vi "PPR_DRIVE_DASH_WRITE.vi"   [LabVIEW 2019]
uses:
  PPR_DRIVE_GLOBALS.vi
  <vilib>/Rock Robotics/Network Tables/NT Write Number.vi
  <vilib>/Rock Robotics/Network Tables/NT Write Numeric Array.vi
  <vilib>/Rock Robotics/WPI/ThirdParty/JAS_Junk/TrajLib/Trajectory_Library.lvlib
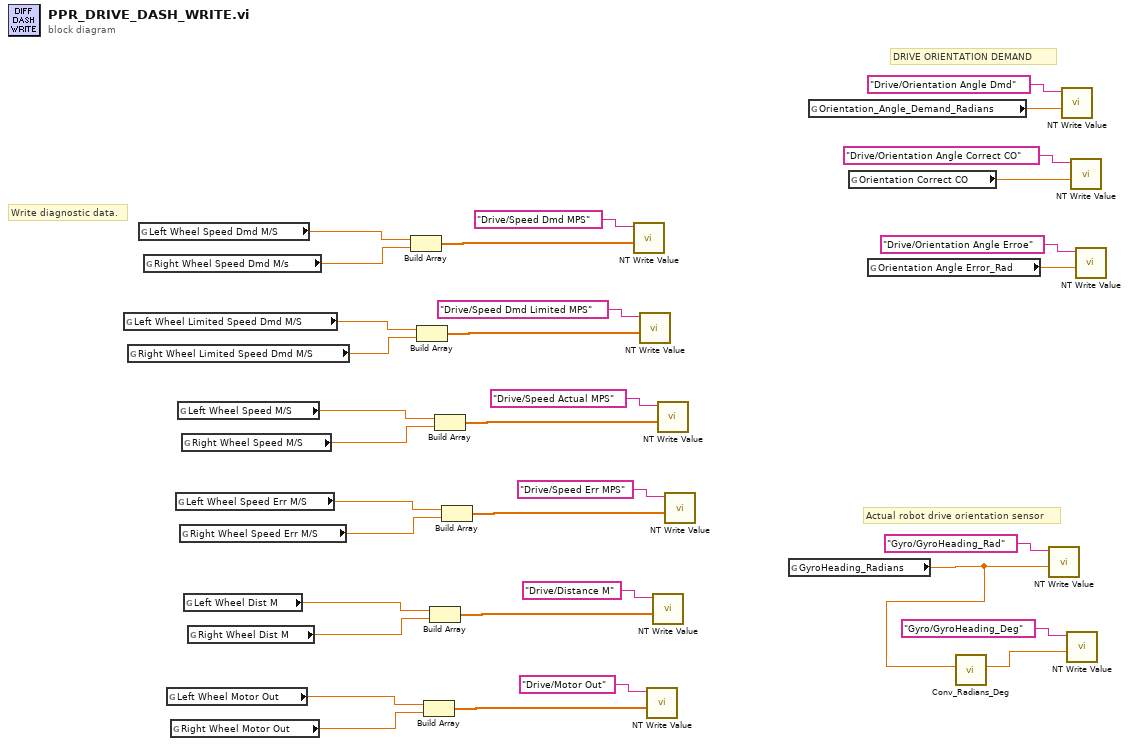
[diagram p0: block diagram]
diagram:
  # "Write diagnostic data."
  # "Actual robot drive orientation sensor"
  # "DRIVE ORIENTATION DEMAND"
  n1 = global read "PPR_DRIVE_GLOBALS.vi" "Left Wheel Limited Speed Dmd M/S"() -> (w19:dbl)
  n2 = global read "PPR_DRIVE_GLOBALS.vi" "Right Wheel Limited Speed Dmd M/S"() -> (w18:dbl)
  n3 = global read "PPR_DRIVE_GLOBALS.vi" "Left Wheel Speed Dmd M/S"() -> (w23:dbl)
  n4 = global read "PPR_DRIVE_GLOBALS.vi" "Right Wheel Speed Dmd M/s"() -> (w22:dbl)
  n5 = global read "PPR_DRIVE_GLOBALS.vi" "Left Wheel Motor Out"() -> (w3:dbl)
  n6 = global read "PPR_DRIVE_GLOBALS.vi" "Right Wheel Motor Out"() -> (w2:dbl)
  n7 = global read "PPR_DRIVE_GLOBALS.vi" "Left Wheel Speed Err M/S"() -> (w11:dbl)
  n8 = global read "PPR_DRIVE_GLOBALS.vi" "Left Wheel Speed M/S"() -> (w15:dbl)
  n9 = global read "PPR_DRIVE_GLOBALS.vi" "Right Wheel Speed Err M/S"() -> (w10:dbl)
  n10 = global read "PPR_DRIVE_GLOBALS.vi" "Right Wheel Speed M/S"() -> (w14:dbl)
  n11 = global read "PPR_DRIVE_GLOBALS.vi" "Left Wheel Dist M"() -> (w7:dbl)
  n12 = global read "PPR_DRIVE_GLOBALS.vi" "Right Wheel Dist M"() -> (w6:dbl)
  n13 = Build Array(w23, w22) -> (w21:dbl[])
  n14 = Build Array(w19, w18) -> (w17:dbl[])
  n15 = Build Array(w3, w2) -> (w1:dbl[])
  n16 = Build Array(w7, w6) -> (w5:dbl[])
  n17 = Build Array(w15, w14) -> (w13:dbl[])
  n18 = Build Array(w11, w10) -> (w9:dbl[])
  n19 = call-poly <vilib>:"NT Write Value.vi"("value"=w21, "name"="Drive/Speed Dmd MPS" ("Name")) -> ()  [unwired: 9 in, 1 out]
  n20 = call-poly <vilib>:"NT Write Value.vi"("value"=w17, "name"="Drive/Speed Dmd Limited MPS" ("Name")) -> ()  [unwired: 9 in, 1 out]
  n21 = call-poly <vilib>:"NT Write Value.vi"("value"=w1, "name"="Drive/Motor Out" ("Name")) -> ()  [unwired: 9 in, 1 out]
  n22 = call-poly <vilib>:"NT Write Value.vi"("value"=w5, "name"="Drive/Distance M" ("Name")) -> ()  [unwired: 9 in, 1 out]
  n23 = call-poly <vilib>:"NT Write Value.vi"("value"=w13, "name"="Drive/Speed Actual MPS" ("Name")) -> ()  [unwired: 9 in, 1 out]
  n24 = call-poly <vilib>:"NT Write Value.vi"("value"=w9, "name"="Drive/Speed Err MPS" ("Name")) -> ()  [unwired: 9 in, 1 out]
  n25 = global read "PPR_DRIVE_GLOBALS.vi" "GyroHeading_Radians"() -> (w24:dbl)
  n26 = global read "PPR_DRIVE_GLOBALS.vi" "Orientation_Angle_Demand_Radians"() -> (w29:dbl)
  n27 = global read "PPR_DRIVE_GLOBALS.vi" "Orientation Correct CO"() -> (w28:dbl)
  n28 = global read "PPR_DRIVE_GLOBALS.vi" "Orientation Angle Error_Rad"() -> (w27:dbl)
  n29 = call <vilib>:"Conv_Radians_Deg.vi"("Radians"=w24) -> ("Degrees"=w25:dbl)  [unwired: 10 in]
  n30 = call-poly <vilib>:"NT Write Value.vi"("value"=w24, "name"="Gyro/GyroHeading_Rad" ("Name")) -> ()  [unwired: 9 in, 1 out]
  n31 = call-poly <vilib>:"NT Write Value.vi"("value"=w29, "name"="Drive/Orientation Angle Dmd" ("Name")) -> ()  [unwired: 9 in, 1 out]
  n32 = call-poly <vilib>:"NT Write Value.vi"("value"=w25, "name"="Gyro/GyroHeading_Deg" ("Name")) -> ()  [unwired: 9 in, 1 out]
  n33 = call-poly <vilib>:"NT Write Value.vi"("value"=w28, "name"="Drive/Orientation Angle Correct CO" ("Name")) -> ()  [unwired: 9 in, 1 out]
  n34 = call-poly <vilib>:"NT Write Value.vi"("value"=w27, "name"="Drive/Orientation Angle Erroe" ("Name")) -> ()  [unwired: 9 in, 1 out]
